vi "slider_outlet_color.vi"(6 "outflow":dbl, 8 "a2":dbl, 9 "A (Crosssection of Tank 2)\n[m²]":dbl, 10 "2g":dbl, 11 "Slide in":refnum<vi>) -> ()   [LabVIEW 2020]
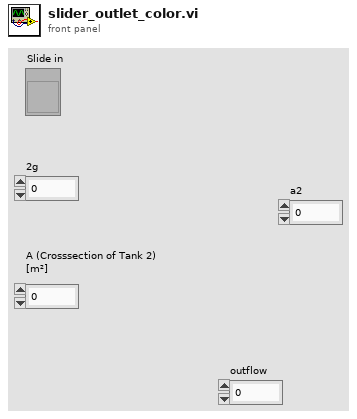
[diagram p1: front panel]
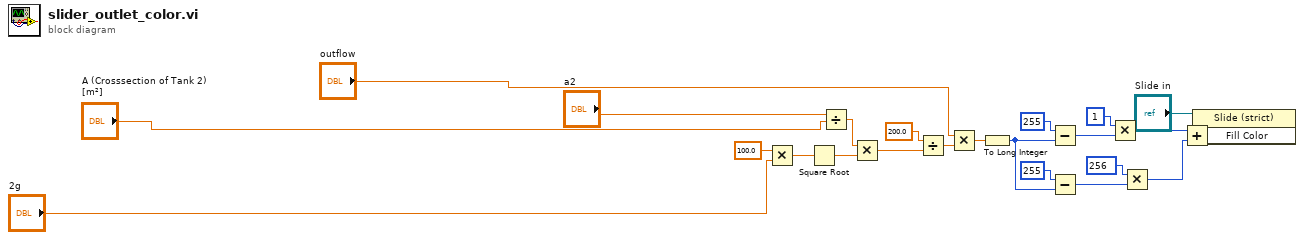
[diagram p0: block diagram]
diagram:
  n1 = Multiply(x=100.0 ("y"), y="2g") -> (x*y=w16:dbl)
  n2 = Square Root(x=w16) -> (sqrt(x)=w17:dbl)
  n3 = Divide(x="a2", y="A (Crosssection of Tank 2)\n[m²]") -> (x/y=w18:dbl)
  n4 = Multiply(x=w18, y=w17) -> (x*y=w19:dbl)
  n5 = Divide(x=200.0, y=w19) -> (x/y=w13:dbl)
  n6 = Multiply(x="outflow", y=w13) -> (x*y=w14:dbl)
  n7 = To Long Integer(number=w14) -> (32bit integer=w10:i32)
  n8 = Subtract(x=255, y=w10) -> (x-y=w8:i32)
  n9 = Subtract(x=255, y=w10) -> (x-y=w11:i32)
  n10 = Multiply(x=1, y=w8) -> (x*y=w3:i32)
  n11 = Multiply(x=256, y=w11) -> (x*y=w4:i32)
  n12 = Add(x=w3, y=w4) -> (x+y=w21:i32)
  n13 = property on="Property Node" class="Slide (strict)"(reference="Slide in", "Fill Color"=w21) -> ()  [unwired: 1 in, 2 out]
